vi "dfd_SCL_ASymFIRm_Odd_CU.vi"(9 "global reset":bool, 10 "output valid":bool, 11 "index":u16) -> (3 "control info":T1)   [LabVIEW 2017]
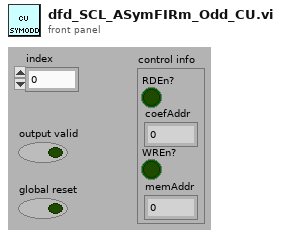
[diagram p1: front panel]
types:
  T1 = cluster{"RDEn?":bool, "coefAddr":u16, "WREn?":bool, "memAddr":u16}
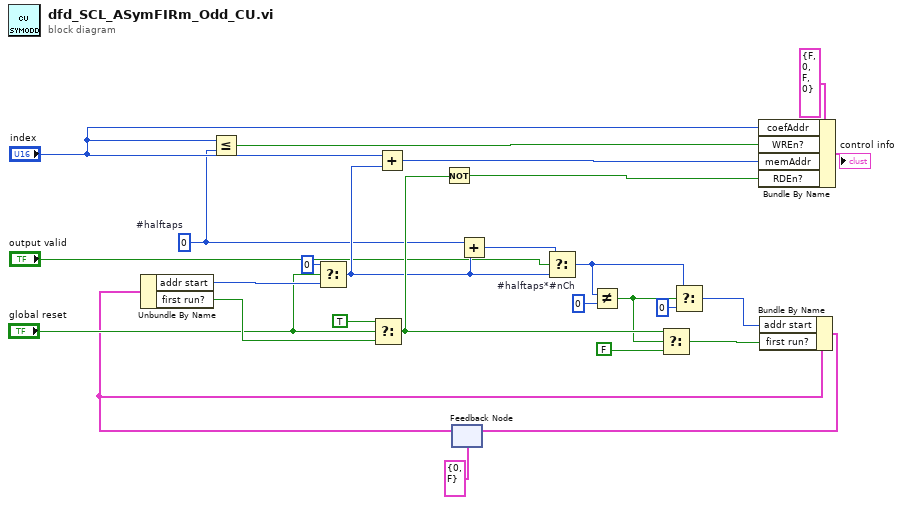
[diagram p0: block diagram]
diagram:
  w14 = u16 0  # #halftaps*#nCh
  w2 = u16 0  # #halftaps
  n1 = Less Or Equal?(x="index", y=w2) -> (x <= y?=w9:bool)
  n2 = feedback #1(cluster{"addr start":u16, "first run?":bool} {"addr start"=0, "first run?"=FALSE} ("states 2")) -> (w5:cluster{"addr start":u16, "first run?":bool})
  n3 = Unbundle By Name(w5) -> ("addr start"=w25:u16, "first run?"=w26:bool)
  n4 = Select(t=u16 0, s="global reset", f=w25) -> (s? t:f=w10:u16)
  n5 = Select(t=TRUE, s="global reset", f=w26) -> (s? t:f=w22:bool)
  n6 = Add(x="index", y=w10) -> (x+y=w8:u16)
  n7 = Not(x=w22) -> (.not. x?=w12:bool)
  n8 = Add(x=w2, y=w10) -> (x+y=w16:u16)
  n9 = Select(t=w16, s="output valid", f=w10) -> (s? t:f=w17:u16)
  n10 = Not Equal?(x=w17, y=w14) -> (x != y?=w19:bool)
  n11 = Select(t=w22, s=w19, f=FALSE ("t")) -> (s? t:f=w24:bool)
  n12 = Select(t=w17, s=w19, f=u16 0) -> (s? t:f=w23:u16)
  n13 = Bundle By Name(cluster=T1 {"RDEn?"=FALSE, "coefAddr"=0, "WREn?"=FALSE, "memAddr"=0} ("control info 2"), "coefAddr"="index", "WREn?"=w9, "memAddr"=w8, "RDEn?"=w12) -> (→"control info":T1)
  n14 = Bundle By Name(cluster=w5, "addr start"=w23, "first run?"=w24) -> (w4:cluster{"addr start":u16, "first run?":bool})
  n15 = feedback-in #1(w4) -> ()
